vi "Verify Acquisition.vi"(8 "error in (no error)":errorcluster, 11 "CCDCamera in":refnum<class "Simulated Camera.lvclass">) -> (0 "error out":errorcluster, 3 "CCDCamera out":refnum<class "Simulated Camera.lvclass">)   [LabVIEW 2018, in "Simulated Camera.lvclass"]
doc: "Verify if the camera is exposing.\n\nIf the exposure still running, the CCD status will be ACTIVE. Otherwise, it will be IDLE"
uses:
  Simulated Camera.lvclass
  Simulated Camera.lvclass/Simulated Camera.ctl
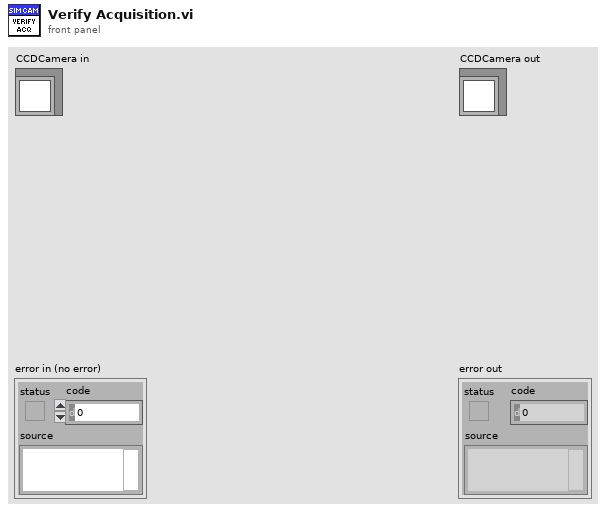
[diagram p1: front panel]
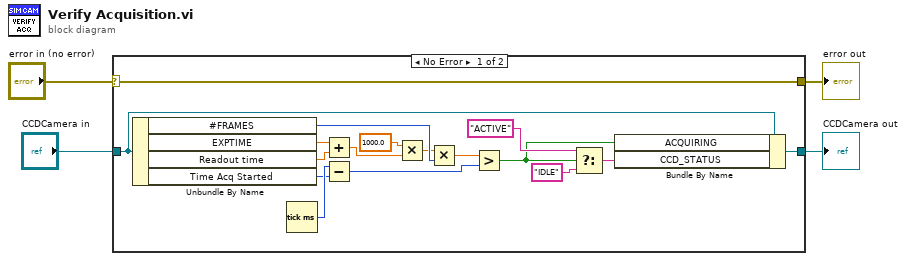
[diagram p0: block diagram]
diagram:
  n1 = case shown="No Error" "error in (no error)" {
    selector: "error in (no error)" -> [w16 w23]
    tunnel: [w16 w23] -> w1
    tunnel: [w11 w22] -> w2
    tunnel: "CCDCamera in" -> [w12 w22]
    frame No Error {
      n2 = Unbundle By Name(w12) -> ("#FRAMES"=w10:u32, "EXPTIME"=w7:dbl, "Readout time"=w8:dbl, "Time Acq Started"=w17:u32)
      n3 = Tick Count (ms)() -> (millisecond timer value=w21:u32)
      n4 = Add(x=w7, y=w8) -> (x+y=w6:dbl)
      n5 = Subtract(x=w21, y=w17) -> (x-y=w20:u32)
      n6 = Multiply(x=1000.0, y=w6) -> (x*y=w5:dbl)
      n7 = Multiply(x=w5, y=w10) -> (x*y=w18:dbl)
      n8 = Greater?(x=w18, y=w20) -> (0:w13:bool)
      n9 = Select(t="ACTIVE", s=w13, f="IDLE") -> (s? t:f=w15:string)
      n10 = Bundle By Name(cluster=w12, "ACQUIRING"=w13, "CCD_STATUS"=w15) -> (w11:refnum<class "Simulated Camera.lvclass">)
    }
    frame Error {
    }
  }
  "error out" <- w1
  "CCDCamera out" <- w2
